vi "AppLauncher.vi"() -> ()   [LabVIEW 2016]
uses:
  <vilib>/JKI/JKI SMO/SMO/Typedefs/SMOState --Enum.ctl
  SMOs/lockin/system.lvclass
  C:/Program Files (x86)/National Instruments/LabVIEW 2016/vi.lib/JKI/JKI SMO/SMO/SMO.lvclass
  SMOs/UI_Main_Test/UI_Main.lvclass
  <vilib>/JKI/JKI SMO/SMO/SMO.lvclass
  SMOs/DAQ/DAQ.lvclass
  SMOs/DAQmx.AI/DAQmx.AI.lvclass
  SMOs/DAQmx.AO/DAQmx.AO.lvclass
  SMOs/DSP/DSP.lvclass
panel:
  out "UI SMO State":T1
  out "System SMO State":T1
  out "error out":errorcluster
  in  "Stop":bool
  # "AppLauncher"
  # "This VI launches the system_backend and UI_frontend.\nIt can run minimized"
  # "For instructions on how to use the JKI State Machine Objects, examples and video tutorials, visit:\nhttp://jki.net/state-machine-objects/\n\nJKI State Machine Objects™\nhttp://jki.net/state-machine-objects/\nCopyright (C) 2005-2015, JKI <info@jki.net>\nALL RIGHTS RESERVED"
  # "should make call directly to lockin"
  # "use network streams to pass data between different computers?\nOr ZeroMQ?\nhave lockin running on different (or same) computers\none is AO/AI\nThe other is lockin DSP"
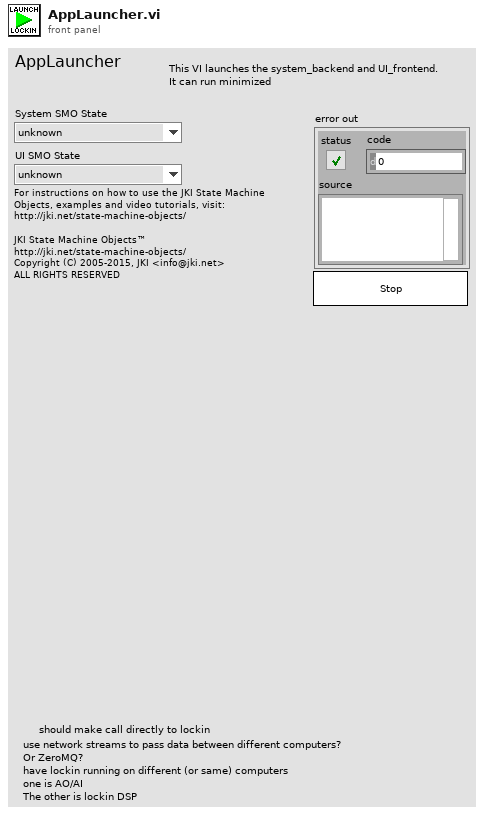
[diagram p1: front panel]
types:
  T1 = typedef "SMO.lvclass/SMOState --Enum.ctl" = enum16{"unknown", "Created", "Started", "Stopped"}
  T2 = typedef "SMO.lvclass/Public Events.ctl" = cluster{"Error":refnum<user-event>, "State":refnum<user-event>, "Reserve State":refnum<user-event>}
  T3 = typedef "system.lvclass/PublicEvents--Cluster.ctl" = cluster{"read":refnum<user-event>, "Write":refnum<user-event>, "lockin_REF_waveform":refnum<user-event>, "lockin_results":refnum<user-event>}
  T4 = cluster{"Event Registration Refnum":refnum<event-registration>}
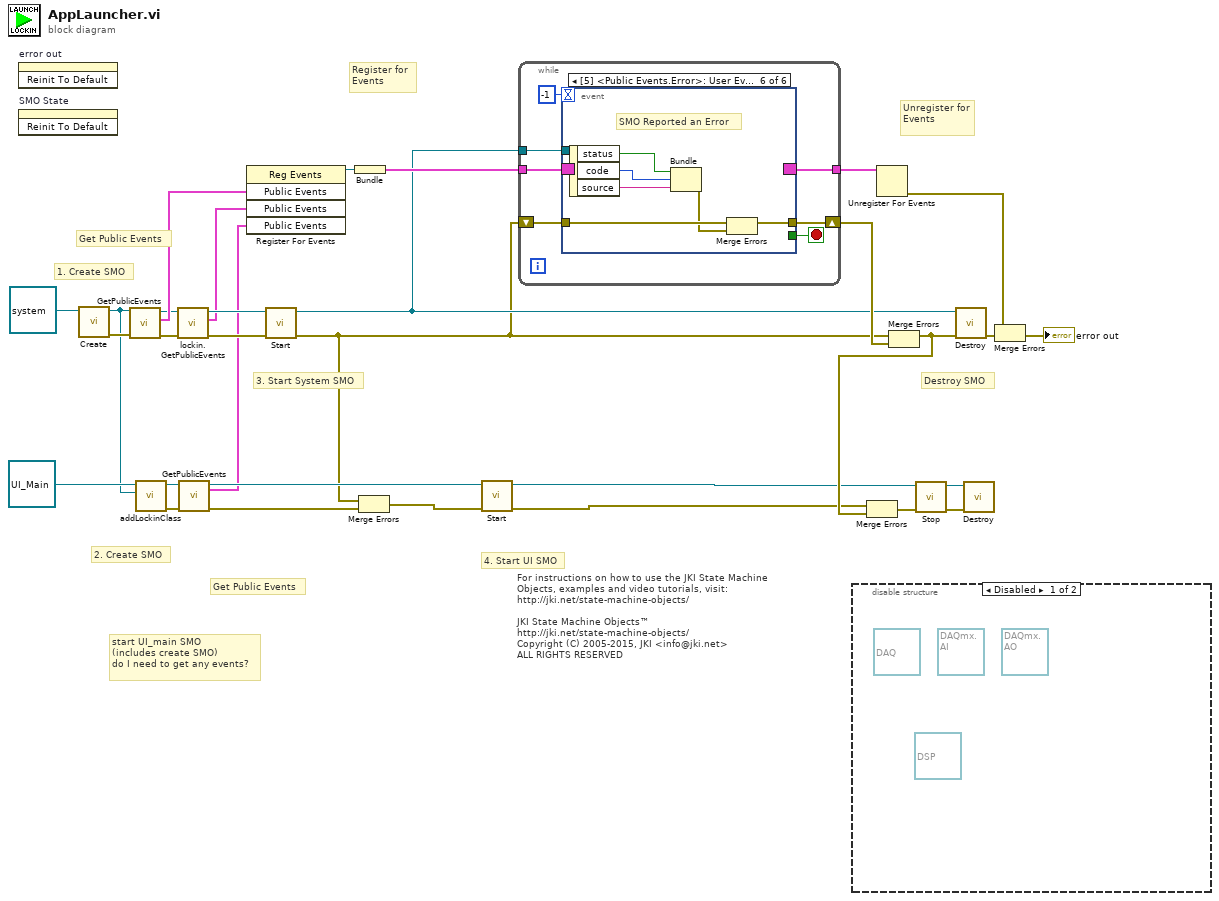
[diagram p0: block diagram]
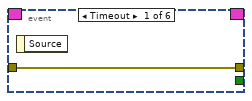
[diagram p3: hidden frame]
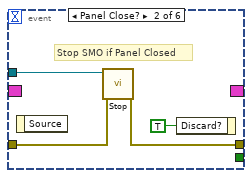
[diagram p4: hidden frame]
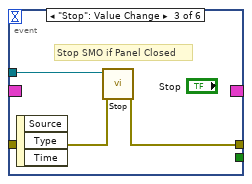
[diagram p5: hidden frame]
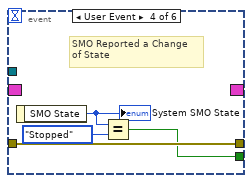
[diagram p6: hidden frame]
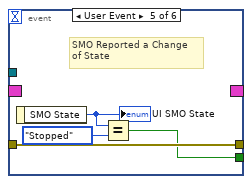
[diagram p7: hidden frame]
diagram:
  # "4. Start UI SMO"
  # "2. Create SMO"
  # "start UI_main SMO\n(includes create SMO)\ndo I need to get any events?"
  # "Get Public Events"
  # "For instructions on how to use the JKI State Machine Objects, examples and video tutorials, visit:\nhttp://jki.net/state-machine-objects/\n\nJKI State Machine Objects™\nhttp://jki.net/state-machine-objects/\nCopyright (C) 2005-2015, JKI <info@jki.net>\nALL RIGHTS RESERVED"
  # "Get Public Events"
  # "3. Start System SMO"
  # "Destroy SMO"
  # "1. Create SMO"
  # "Unregister for Events"
  # "Register for Events"
  n1 = invoke on="error out" class="Clust (strict)" method="Reinit To Default"() -> ()  [unwired: 3 in, 3 out]
  n2 = invoke on="SMO State" class="Enum (strict)" method="Reinit To Default"() -> ()  [unwired: 3 in, 3 out]
  n3 = call <vilib>:"Create.vi"("SMO"=refnum<class "system.lvclass"> refnum ("SMO.Template.lvclass")) -> ("error out"=w25:errorcluster, "SMO out"=w11:refnum<class "system.lvclass">)  [unwired: 8 in, 1 out]
  n4 = call <vilib>:"GetPublicEvents.vi"("error in (no error)"=w25, "SMO"=w11) -> ("error out"=w10:errorcluster, "Public Events"=w24:T2, "SMO out"=w9:refnum<class "system.lvclass">)  [unwired: 7 in]
  n5 = call "addLockinClass.vi"("system.lvclass"=w11, "UI_Main in"=refnum<class "UI_Main.lvclass"> refnum ("UI_Main.lvclass")) -> ("error out"=w13:errorcluster, "UI_Main out"=w14:refnum<class "UI_Main.lvclass">)  [unwired: 8 in]
  n6 = call "lockin.GetPublicEvents.vi"("error in (no error)"=w10, "lockin"=w9) -> ("error out"=w7:errorcluster, "Public Events"=w2:T3, "lockin out"=w8:refnum<class "system.lvclass">)  [unwired: 7 in]
  n7 = call <vilib>:"GetPublicEvents.vi"("error in (no error)"=w13, "SMO"=w14) -> ("error out"=w5:errorcluster, "Public Events"=w1:T2, "SMO out"=w6:refnum<class "UI_Main.lvclass">)  [unwired: 7 in]
  n8 = register-events(w24, w2, w1) -> (reference out=w23:refnum<event-registration>)  [unwired: 2 in, 1 out]
  n9 = call <vilib>:"Start.vi"("error in (no error)"=w7, "SMO"=w8) -> ("error out"=w4:errorcluster, "SMO out"=w22:refnum<class "system.lvclass">)  [unwired: 8 in]
  n10 = Bundle("Event Registration Refnum"=w23) -> (w30:T4)  [unwired: 1 in]
  n11 = Merge Errors(w4, w5) -> (w3:errorcluster)
  n12 = call <vilib>:"Start.vi"("error in (no error)"=w3, "SMO"=w6) -> ("error out"=w17:errorcluster, "SMO out"=w16:refnum<class "UI_Main.lvclass">)  [unwired: 8 in]
  n13 = while {
    shift-right: [w37] -> w29
    shift-left: w4 -> [w36]
    tunnel: w30 -> [w35]
    tunnel: [w34] -> w31
    tunnel: w22 -> [w33]
    stop <- w38 stop-if-true
    n14 = event shown="[5] <Public Events.Error>: User Event" {
      selector: w35 -> [_ _ _ _ _ _]
      dyn-events: [_ _ _ _ _ _] -> w34
      timeout: -1 -> [_ _ _ _ _ _]
      tunnel: [_ _ _ w47 w51 _] -> w38
      tunnel: w33 -> [_ w43 w46 _ _ _]
      tunnel: [w39 w42 w45 w50 w54 w58] -> w37
      tunnel: w36 -> [w39 w41 w44 w50 w54 w56]
      event Timeout {
        n15 = event-data() -> ()  [unwired: 1 in, 1 out]
      }
      event Panel Close? {
        # "Stop SMO if Panel Closed"
        n16 = event-data() -> ()  [unwired: 1 in, 1 out]
        n17 = call <vilib>:"Stop.vi"("error in (no error)"=w41, "SMO"=w43) -> ("error out"=w42:errorcluster)  [unwired: 8 in, 1 out]
        n18 = event-data("Discard?"=TRUE ("OK")) -> ()  [unwired: 1 in, 1 out]
      }
      event "Stop": Value Change {
        # "Stop SMO if Panel Closed"
        n19 = event-data() -> ()  [unwired: 1 in, 3 out]
        n20 = call <vilib>:"Stop.vi"("error in (no error)"=w44, "SMO"=w46) -> ("error out"=w45:errorcluster)  [unwired: 8 in, 1 out]
      }
      event User Event {
        # "SMO Reported a Change\nof State"
        n21 = event-data() -> ("SMO State"=w49:T1)  [unwired: 1 in]
        "System SMO State" <- w49
        n22 = Equal?(x=w49, y=SMOState_--Enum."Stopped") -> (x = y?=w47:bool)
      }
      event User Event {
        # "SMO Reported a Change\nof State"
        n23 = event-data() -> ("SMO State"=w53:T1)  [unwired: 1 in]
        "UI SMO State" <- w53
        n24 = Equal?(x=w53, y=SMOState_--Enum."Stopped") -> (x = y?=w51:bool)
      }
      event User Event {
        # "SMO Reported an Error"
        n25 = event-data() -> ("status"=w57:bool, "code"=w60:i32, "source"=w59:string)  [unwired: 1 in]
        n26 = Bundle("status"=w57, "code"=w60, "source"=w59) -> (w55:errorcluster)  [unwired: 1 in]
        n27 = Merge Errors(w56, w55) -> (w58:errorcluster)
      }
    }
  }
  n28 = disable-structure shown="Disabled" {
    frame Disabled {
      (unwired) refnum<class "DSP.lvclass"> refnum ("DSP.lvclass")
      (unwired) refnum<class "DAQmx.AO.lvclass"> refnum ("DAQmx.AO.lvclass")
      (unwired) refnum<class "DAQmx.AI.lvclass"> refnum ("DAQmx.AI.lvclass")
      (unwired) refnum<class "DAQ.lvclass"> refnum ("DAQ.lvclass")
    }
    frame Enabled {
    }
  }
  n29 = Unregister For Events(event registration refnum=w31) -> (error out=w28:errorcluster)  [unwired: 1 in]
  n30 = Merge Errors(w4, w29) -> (w19:errorcluster)
  n31 = Merge Errors(w17, w19) -> (w18:errorcluster)
  n32 = call <vilib>:"Stop.vi"("error in (no error)"=w18, "SMO"=w16) -> ("error out"=w20:errorcluster, "SMO out"=w21:refnum<class "UI_Main.lvclass">)  [unwired: 8 in]
  n33 = call <vilib>:"Destroy.vi"("error in (no error)"=w19, "SMO"=w22) -> ("error out"=w26:errorcluster)  [unwired: 9 in]
  n34 = call <vilib>:"Destroy.vi"("error in (no error)"=w20, "SMO"=w21) -> ()  [unwired: 9 in, 1 out]
  n35 = Merge Errors(w28, w26) -> (→"error out":errorcluster)
